vi "Gen_Photon_Events.vi"() -> (2 "Channel":dbl, 3 "Time":u64)   [LabVIEW 2023]
uses:
  <vilib>/numeric/Random Number (Range) U64.vi
  <vilib>/numeric/sub_Random U32.vi
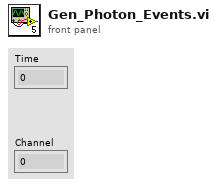
[diagram p1: front panel]
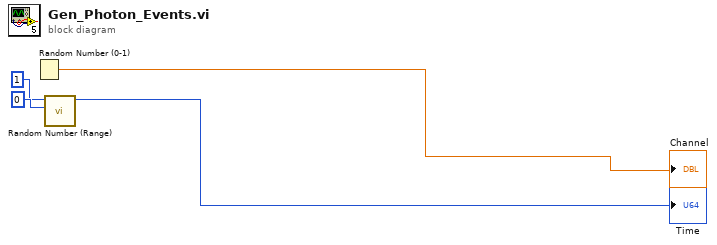
[diagram p0: block diagram]
diagram:
  n1 = Random Number (0-1)() -> (number: 0 to 1=→"Channel":dbl)
  n2 = call-poly <vilib>:"Random Number (Range).vi"("lower bound (0)"=u64 0, "upper bound (100)"=u64 1) -> ("number"=→"Time":u64)  [unwired: 9 in]
